vi "VisualInspectionEBAY.vi"(8 "error in (no error)":errorcluster, 11 "TableRef":refnum<vi>) -> (0 "error out":errorcluster, 2 "VisualInspectionResult":bool)   [LabVIEW 2017]
panel:
  in  "13":dbl
  in  "17.1":dbl
  in  "16.3":dbl
  in  "16.2":dbl
  in  "16.1":dbl
  in  "15.2":dbl
  in  "15.1":dbl
  in  "14.1":dbl
  in  "12.4":dbl
  in  "12.3":dbl
  in  "12.2":dbl
  in  "12.1":dbl
  in  "11.1":dbl
  in  "18":bool
  in  "10.2":bool
  in  "10.1":bool
  in  "Cancel Button":bool
  in  "OK Button":bool
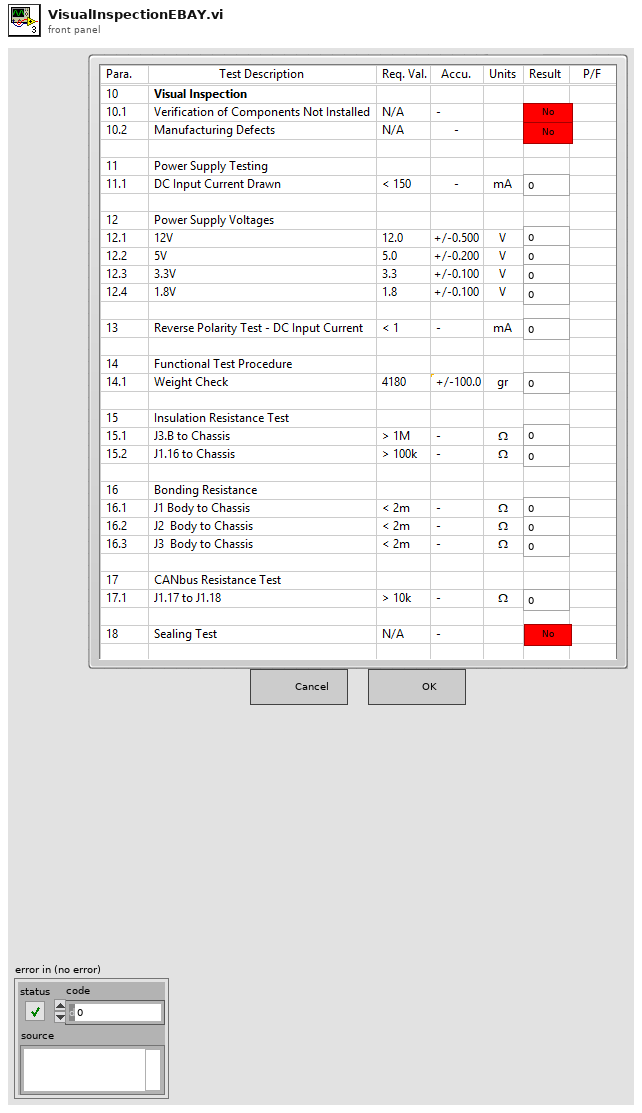
[diagram p1: front panel]
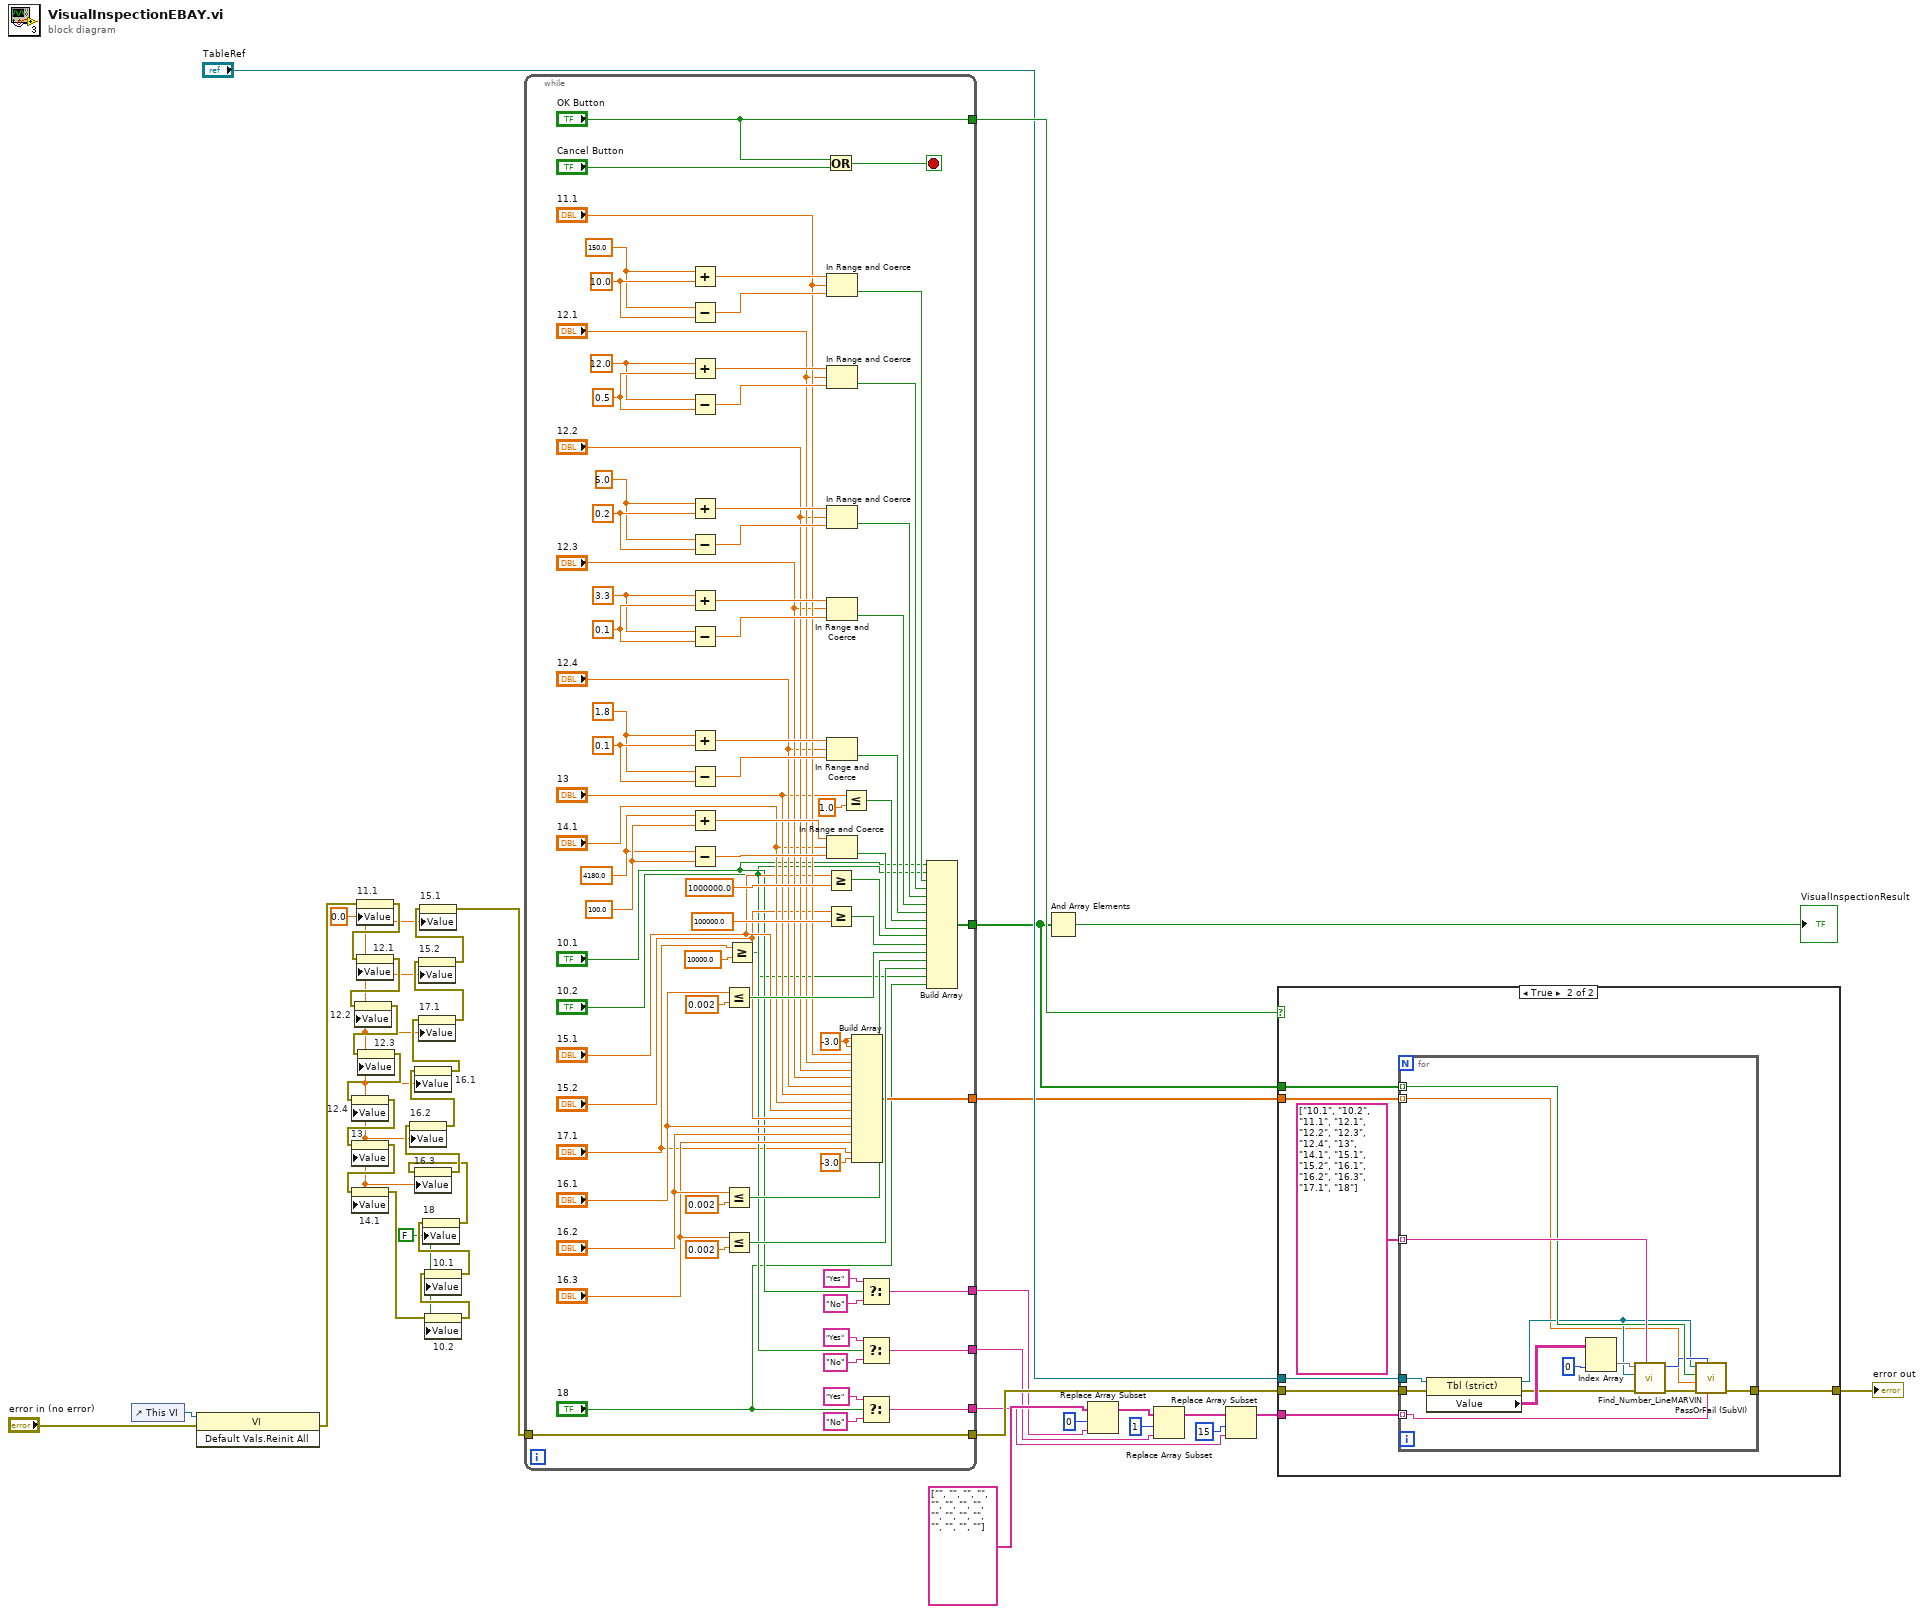
[diagram p0: block diagram]
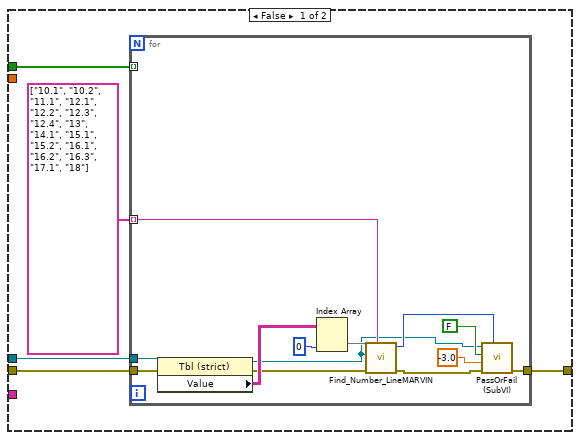
[diagram p2: hidden frame]
diagram:
  w1 = FALSE ("18")
  w6 = 0.0 ("11.1")
  n1 = control-ref of="This VI"() -> (w35:refnum<vi>)
  n2 = invoke class="VI" method="Default Vals.Reinit All"(reference=w35, error in="error in (no error)") -> (error out=w7:errorcluster)  [unwired: 1 in, 2 out]
  n3 = property on="11.1" class="DigNum (strict)"(error in=w7, "Value"=w6) -> (error out=w19:errorcluster)  [unwired: 1 in, 1 out]
  n4 = property on="12.1" class="DigNum (strict)"(error in=w19, "Value"=w6) -> (error out=w18:errorcluster)  [unwired: 1 in, 1 out]
  n5 = property on="12.2" class="DigNum (strict)"(error in=w18, "Value"=w6) -> (error out=w17:errorcluster)  [unwired: 1 in, 1 out]
  n6 = property on="12.3" class="DigNum (strict)"(error in=w17, "Value"=w6) -> (error out=w16:errorcluster)  [unwired: 1 in, 1 out]
  n7 = property on="12.4" class="DigNum (strict)"(error in=w16, "Value"=w6) -> (error out=w15:errorcluster)  [unwired: 1 in, 1 out]
  n8 = property on="13" class="DigNum (strict)"(error in=w15, "Value"=w6) -> (error out=w14:errorcluster)  [unwired: 1 in, 1 out]
  n9 = property on="14.1" class="DigNum (strict)"(error in=w14, "Value"=w6) -> (error out=w5:errorcluster)  [unwired: 1 in, 1 out]
  n10 = property on="10.2" class="Bool (strict)"(error in=w5, "Value"=w1) -> (error out=w4:errorcluster)  [unwired: 1 in, 1 out]
  n11 = property on="10.1" class="Bool (strict)"(error in=w4, "Value"=w1) -> (error out=w3:errorcluster)  [unwired: 1 in, 1 out]
  n12 = property on="18" class="Bool (strict)"(error in=w3, "Value"=w1) -> (error out=w2:errorcluster)  [unwired: 1 in, 1 out]
  n13 = property on="16.3" class="DigNum (strict)"(error in=w2, "Value"=w6) -> (error out=w13:errorcluster)  [unwired: 1 in, 1 out]
  n14 = property on="16.2" class="DigNum (strict)"(error in=w13, "Value"=w6) -> (error out=w12:errorcluster)  [unwired: 1 in, 1 out]
  n15 = property on="16.1" class="DigNum (strict)"(error in=w12, "Value"=w6) -> (error out=w11:errorcluster)  [unwired: 1 in, 1 out]
  n16 = property on="17.1" class="DigNum (strict)"(error in=w11, "Value"=w6) -> (error out=w10:errorcluster)  [unwired: 1 in, 1 out]
  n17 = property on="15.2" class="DigNum (strict)"(error in=w10, "Value"=w6) -> (error out=w9:errorcluster)  [unwired: 1 in, 1 out]
  n18 = property on="15.1" class="DigNum (strict)"(error in=w9, "Value"=w6) -> (error out=w8:errorcluster)  [unwired: 1 in, 1 out]
  n19 = while {
    tunnel: w8 -> [w111]
    tunnel: [w113] -> w32
    tunnel: ["OK Button"] -> w38
    tunnel: [w111] -> w37
    tunnel: [w66] -> w30
    tunnel: [w45] -> w23
    tunnel: [w44] -> w22
    tunnel: [w43] -> w21
    stop <- w114 stop-if-true
    w67 = -3.0 ("element")
    w90 = 0.5 ("y")
    w92 = 0.2 ("y")
    w94 = 0.1 ("y")
    w96 = 0.1 ("y")
    w98 = 100.0 ("y")
    w88 = 10.0 ("y")
    w97 = 4180.0 ("y")
    w95 = 1.8 ("y")
    w93 = 3.3 ("y")
    w91 = 5.0 ("y")
    w89 = 12.0 ("y")
    w87 = 150.0 ("y")
    n20 = Add(x=w87, y=w88) -> (x+y=w99:dbl)
    n21 = Subtract(x=w87, y=w88) -> (x-y=w100:dbl)
    n22 = Add(x=w89, y=w90) -> (x+y=w101:dbl)
    n23 = Subtract(x=w89, y=w90) -> (x-y=w102:dbl)
    n24 = Add(x=w91, y=w92) -> (x+y=w103:dbl)
    n25 = Subtract(x=w91, y=w92) -> (x-y=w104:dbl)
    n26 = Add(x=w93, y=w94) -> (x+y=w105:dbl)
    n27 = Subtract(x=w93, y=w94) -> (x-y=w106:dbl)
    n28 = Add(x=w95, y=w96) -> (x+y=w107:dbl)
    n29 = Subtract(x=w95, y=w96) -> (x-y=w108:dbl)
    n30 = Add(x=w97, y=w98) -> (x+y=w109:dbl)
    n31 = Subtract(x=w97, y=w98) -> (x-y=w110:dbl)
    n32 = Less Or Equal?(x="16.1", y=0.002) -> (x <= y?=w70:bool)
    n33 = Less Or Equal?(x="16.2", y=0.002) -> (x <= y?=w69:bool)
    n34 = Less Or Equal?(x="16.3", y=0.002) -> (x <= y?=w68:bool)
    n35 = Greater Or Equal?(x="17.1", y=10000.0) -> (x >= y?=w41:bool)
    n36 = Or(x="OK Button", y="Cancel Button") -> (x .or. y?=w114:bool)
    n37 = Greater Or Equal?(x="15.1", y=1000000.0) -> (x >= y?=w72:bool)
    n38 = Greater Or Equal?(x="15.2", y=100000.0) -> (x >= y?=w71:bool)
    n39 = In Range and Coerce(upper limit=w99, x="11.1", lower limit=w100) -> (In Range?=w79:bool)  [unwired: 1 out]
    n40 = In Range and Coerce(upper limit=w101, x="12.1", lower limit=w102) -> (In Range?=w78:bool)  [unwired: 1 out]
    n41 = In Range and Coerce(upper limit=w103, x="12.2", lower limit=w104) -> (In Range?=w77:bool)  [unwired: 1 out]
    n42 = In Range and Coerce(upper limit=w105, x="12.3", lower limit=w106) -> (In Range?=w76:bool)  [unwired: 1 out]
    n43 = In Range and Coerce(upper limit=w107, x="12.4", lower limit=w108) -> (In Range?=w75:bool)  [unwired: 1 out]
    n44 = In Range and Coerce(upper limit=w109, x="14.1", lower limit=w110) -> (In Range?=w73:bool)  [unwired: 1 out]
    n45 = Less Or Equal?(x="13", y=1.0) -> (x <= y?=w74:bool)
    n46 = Build Array(w67, w67, "11.1", "12.1", "12.2", "12.3", "12.4", "13", "14.1", "15.1", "15.2", "16.1", "16.2", "16.3", "17.1", -3.0 ("element")) -> (w66:dbl[])
    n47 = Select(t="Yes", s="10.1", f="No") -> (s? t:f=w43:string)
    n48 = Select(t="Yes", s="10.2", f="No") -> (s? t:f=w44:string)
    n49 = Select(t="Yes", s="18", f="No") -> (s? t:f=w45:string)
    n50 = Build Array("10.1", "10.2", w79, w78, w77, w76, w75, w74, w73, w72, w71, w70, w69, w68, w41, "18") -> (w113:bool[])
  }
  n51 = And Array Elements(Boolean array=w32) -> (logical AND=→"VisualInspectionResult":bool)
  n52 = Replace Array Subset(array=string[] ["", "", "", "", "", "", "", "", "", "", "", "", "", "", "", ""], new element=w21, index=0) -> (w28:string[])
  n53 = Replace Array Subset(array=w28, new element=w22, index=1) -> (w27:string[])
  n54 = Replace Array Subset(array=w27, new element=w23, index=15) -> (w20:string[])
  n55 = case shown="True" w38 {
    tunnel: w32 -> [w120 w140]
    tunnel: w37 -> [w119 w139]
    tunnel: [w118 w138] -> w33
    tunnel: "TableRef" -> [w117 w137]
    tunnel: w30 -> [_ w135]
    tunnel: w20 -> [_ w134]
    frame False {
      n56 = for {
        tunnel: string[] ["10.1", "10.2", "11.1", "12.1", "12.2", "12.3", "12.4", "13", "14.1", "15.1", "15.2", "16.1", "16.2", "16.3", "17.1", "18"] ("Array 4") -> [w129] mode=indexing
        tunnel: w120 -> [_] mode=indexing
        tunnel: w119 -> [w126]
        tunnel: [w125] -> w118
        tunnel: w117 -> [w124]
        n57 = property class="Tbl (strict)"(reference=w124, error in=w126) -> (reference out=w122:refnum<vi>, error out=w130:errorcluster, "Value"=w133:string[][])
        n58 = Index Array(array=w133, index (col)=0 ("disabled index (col)")) -> (element=w131:string[])  [unwired: 1 in]
        n59 = call "Find_Number_LineMARVIN.vi"("Test Paragraph"=w129, "error in"=w130, "TableIn"=w122, "Row Headers[]"=w131) -> ("error out"=w128:errorcluster, "Line number"=w127:i32)  [unwired: 1 in, 2 out]
        n60 = call "PassOrFail (SubVI).vi"("index (row)"=w127, "error in (no error)"=w128, "Data in"=-3.0, "Pass?Fail"=FALSE ("Boolean"), "Table in"=w122) -> ("error out"=w125:errorcluster)  [unwired: 6 in]
      }
    }
    frame True {
      n61 = for {
        tunnel: string[] ["10.1", "10.2", "11.1", "12.1", "12.2", "12.3", "12.4", "13", "14.1", "15.1", "15.2", "16.1", "16.2", "16.3", "17.1", "18"] ("Array 4") -> [w150] mode=indexing
        tunnel: w140 -> [w148] mode=indexing
        tunnel: w139 -> [w146]
        tunnel: [w145] -> w138
        tunnel: w137 -> [w144]
        tunnel: w135 -> [w142] mode=indexing
        tunnel: w134 -> [w141] mode=indexing
        n62 = property class="Tbl (strict)"(reference=w144, error in=w146) -> (reference out=w143:refnum<vi>, error out=w151:errorcluster, "Value"=w154:string[][])
        n63 = Index Array(array=w154, index (col)=0 ("disabled index (col)")) -> (element=w152:string[])  [unwired: 1 in]
        n64 = call "Find_Number_LineMARVIN.vi"("Test Paragraph"=w150, "error in"=w151, "TableIn"=w143, "Row Headers[]"=w152) -> ("error out"=w149:errorcluster, "Line number"=w147:i32)  [unwired: 1 in, 2 out]
        n65 = call "PassOrFail (SubVI).vi"("String Res"=w141, "index (row)"=w147, "error in (no error)"=w149, "Data in"=w142, "Pass?Fail"=w148, "Table in"=w143) -> ("error out"=w145:errorcluster)  [unwired: 5 in]
      }
    }
  }
  "error out" <- w33
